vi "Inverse FHT PtByPt.vi"(2 "initialize":bool, 3 "sample length":i32=100, 5 "x":dbl format="%0.2f") -> (0 "error":i32, 1 "Inverse Hartley{X}":dbl[](array[numeric]))   [LabVIEW 2020, in "NI_PtbyPt.lvlib"]
doc: "Computes the inverse fast Hartley transform of the set of input data points specified by <B>sample length</B>."
uses:
  <vilib>/ptbypt/NI_PtbyPt.lvlib
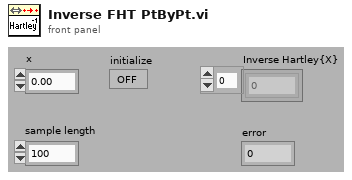
[diagram p1: front panel]
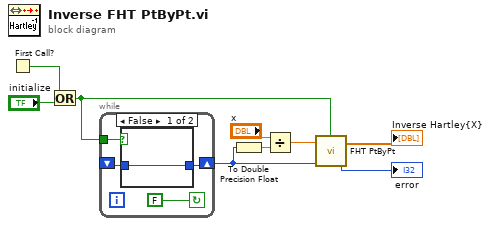
[diagram p0: block diagram]
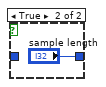
[diagram p2: hidden frame]
diagram:
  n1 = First Call?() -> (First Call?: T/F=w3:bool)
  n2 = Or(x=w3, y="initialize") -> (x .or. y?=w2:bool)
  n3 = while {
    shift-left: _ -> [w11]
    shift-right: [w12] -> w1
    tunnel: w2 -> [w13]
    stop <- FALSE continue-if-true
    n4 = case shown="False" w13 {
      tunnel: [w14 "sample length"] -> w12
      tunnel: w11 -> [w14 _]
      frame False {
      }
      frame True {
      }
    }
  }
  n5 = To Double Precision Float(number=w1) -> (double precision float=w5:dbl)
  n6 = Divide(x="x", y=w5) -> (x/y=w8:dbl)
  n7 = call <vilib>:"FHT PtByPt.vi"("initialize"=w2, "sample length"=w1, "x"=w8) -> ("error"=→"error":i32, "Hartley{X}"=→"Inverse Hartley{X}":dbl[])  [unwired: 1 in]
